vi "Convert TDMS File To No DAQmx Raw 2012 NIVerified.vi"() -> ()   [LabVIEW 2017]
doc: "Open a TDMS file with DQAmxRaw data in it, write all of the data to a new file. The DAQmxRaw datatype is used for high throughput data file writing. Raw ADC Data is stored with scaling factors in the DAQmxRaw datatype. The decoding information for this datatype is not provided by NI in the tdms documentation at: http://zone.ni.com/devzone/cda/tut/p/id/5696. This VI demonstrates how a simple VI can be used to open a TDMS file which contains data in the DAQmxRaw data type and write it to another file (this operation converts the data in the file to the supported data types available to users in the TDMS documentation).\n\nThis will convert DAQmx Raw data which is problematic for reading with other tools (http://www.mathworks.com/matlabcentral/fileexchange/44206-converttdms-v10)."
panel:
  out "Error":errorcluster
  in  "Convert":bool
  in  "Stop":bool
  in  "File With Raw DAQmx":path
  # "Overview: Very simple utility to read in a TDMS file and the write out data to a new TDMS file (which does not use the DAQmx Raw Data type).\nRequirements: LabVIEW 2012 (or compatible)\nInstructions:\n1. Run the VI.\n2. Select File to be converted.\n3. Copy File name from above and change or append to name.\n4. Press OK to convert button."
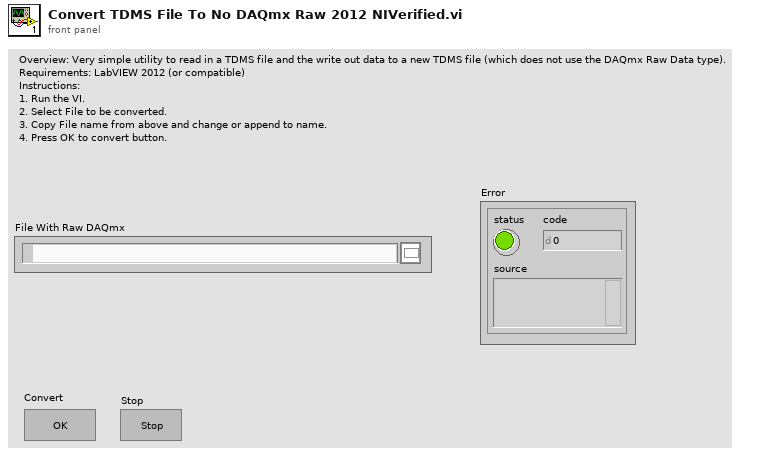
[diagram p1: front panel]
types:
  T1 = enum16{"open", "open or create", "create or replace", "create", "open (read-only)"}
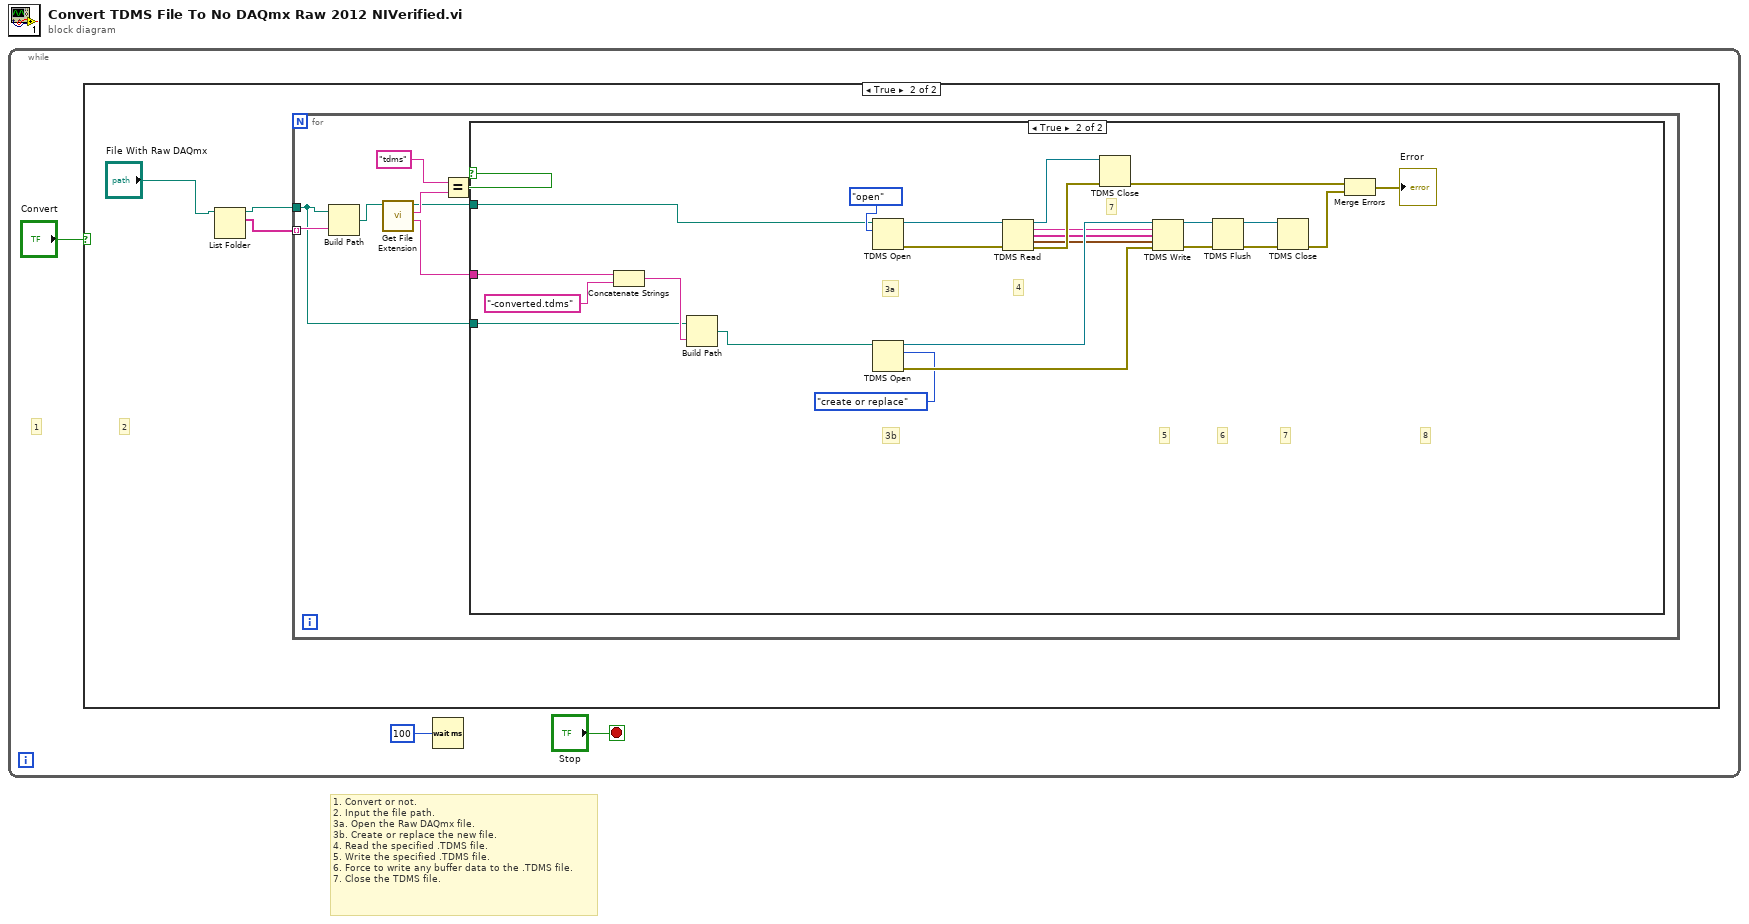
[diagram p0: block diagram]
diagram:
  # "1. Convert or not.\n2. Input the file path.\n3a. Open the Raw DAQmx file.\n3b. Create or replace the new file.\n4. Read the specified .TDMS file.\n5. Write the specified .TDMS file.\n6. Force to write any buffer data to the .TDMS file. \n7. Close the TDMS file."
  n1 = while {
    stop <- "Stop" stop-if-true
    # "1"
    n2 = case shown="True" "Convert" {
      frame False {
      }
      frame True {
        # "2"
        n3 = List Folder(path="File With Raw DAQmx") -> (path out=w4:path, filenames=w5:string[])  [unwired: 3 in, 2 out]
        n4 = for {
          tunnel: w5 -> [w14] mode=indexing
          tunnel: w4 -> [w7]
          n5 = Build Path(base path=w7, name or relative path=w14) -> (appended path=w13:path)
          n6 = call <vilib>:"Get File Extension.vi"("file"=w13) -> ("filename without extension"=w8:string, "lowercase file extension"=w12:string, "dup file"=w9:path)  [unwired: 6 in, 2 out]
          n7 = Equal?(x="tdms", y=w12) -> (x = y?=w10:bool)
          n8 = case shown="True" w10 {
            tunnel: w9 -> [_ w20]
            tunnel: w8 -> [_ w18]
            tunnel: w7 -> [_ w15]
            frame False {
            }
            frame True {
              # "3a"
              # "8"
              # "7"
              # "6"
              # "5"
              # "7"
              # "4"
              # "3b"
              n9 = Concatenate Strings(w18, "-converted.tdms" ("name or relative path")) -> (w16:string)
              n10 = Build Path(base path=w15, name or relative path=w16) -> (appended path=w19:path)
              n11 = TDMS Open(10:T1."open" ("operation (0:open)"), 11:w20) -> (0:w27:errorcluster, 3:w26:refnum<k34>)  [unwired: 5 in]
              n12 = TDMS Open(10:T1."create or replace" ("operation (0:open)"), 11:w19) -> (0:w35:errorcluster, 3:w28:refnum<k34>)  [unwired: 5 in]
              n13 = TDMS Read(0:w26, 11:w27) -> (4:w30:refnum<k34>, 6:w23:string, 8:w24:string[], 10:w25:waveform(dbl)[], 15:w29:errorcluster)  [unwired: 6 in, 1 out]
              n14 = TDMS Close(8:w29, 11:w30) -> (0:w36:errorcluster)  [unwired: 1 out]
              n15 = TDMS Write(0:w28, 5:w23, 7:w24, 9:w25, 11:w35) -> (4:w32:refnum<k34>, 15:w31:errorcluster)  [unwired: 1 in, 2 out]
              n16 = TDMS Flush(4:w31, 7:w32) -> (0:w33:errorcluster, 3:w34:refnum<k34>)
              n17 = TDMS Close(8:w33, 11:w34) -> (0:w37:errorcluster)  [unwired: 1 out]
              n18 = Merge Errors(w36, w37) -> (→"Error":errorcluster)
            }
          }
        }
      }
    }
    n19 = Wait (ms)(milliseconds to wait=u32 100 ("millisecond multiple")) -> ()  [unwired: 1 out]
  }
